vi "Read access time.vi"(8 "error in (no error)":errorcluster, 11 "file attributes in":refnum<class "File Attributes.lvclass">) -> (0 "error out":errorcluster, 2 "access time":timestamp, 3 "file attributes out":refnum<class "File Attributes.lvclass">)   [LabVIEW 2020, in "NI_SFTP.lvlib" / "File Attributes.lvclass"]
doc: "Reads the access time stored in this File Attributes object, returning a LabVIEW timestamp.\n\nThis property may not always be populated by SFTP VIs. If it does not exist, an error is returned."
uses:
  <vilib>/net/SFTP/File Attributes/File Attributes.lvclass
  <vilib>/net/SFTP/File Attributes/File Attributes.lvclass/File Attributes.ctl
  <vilib>/Utility/error.llb/Error Cluster From Error Code.vi
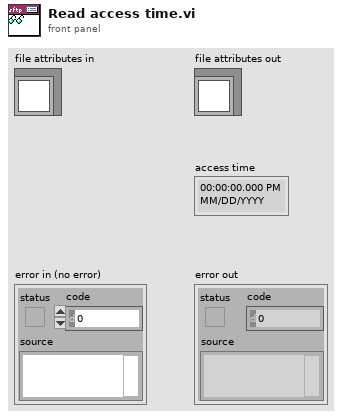
[diagram p1: front panel]
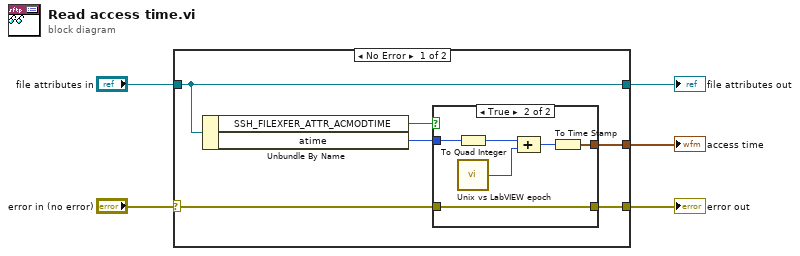
[diagram p0: block diagram]
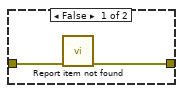
[diagram p2: hidden frame]
diagram:
  n1 = case shown="No Error" "error in (no error)" {
    selector: "error in (no error)" -> [w7 w20]
    tunnel: [w6 w20] -> w4
    tunnel: [w10 w21] -> w2
    tunnel: "file attributes in" -> [w10 w21]
    tunnel: [w9 _] -> w1
    frame No Error {
      n2 = Unbundle By Name(w10) -> ("SSH_FILEXFER_ATTR_ACMODTIME"=w8:bool, "atime"=w11:u32)
      n3 = case shown="True" w8 {
        tunnel: w11 -> [_ w18]
        tunnel: [_ w15] -> w9
        tunnel: w7 -> [w13 w14]
        tunnel: [w12 w14] -> w6
        frame False {
          n4 = call <vilib>:"Report item not found.vi"("error in (no error)"=w13) -> ("error out"=w12:errorcluster)  [unwired: 10 in]
        }
        frame True {
          n5 = To Quad Integer(1:w18) -> (0:w17:i64)
          n6 = call <vilib>:"Unix vs LabVIEW epoch.vi"() -> ("seconds from 1904-01-01 to 1970-01-01"=w16:i64)
          n7 = Compound Arithmetic op=ADD(w17, w16) -> (w19:i64)
          n8 = To Time Stamp(1:w19) -> (0:w15:timestamp)
        }
      }
    }
    frame Error {
    }
  }
  "error out" <- w4
  "file attributes out" <- w2
  "access time" <- w1
